vi "View DI param_1.vi"(7 "ActivateDIView":bool, 9 "DI":T1, 10 "DI_State":T3[](array[typedef]), 11 "DI":bool[](array[boolean])) -> (2 "Reread out":bool)   [LabVIEW 2019, in "Inputs.lvlib"]
uses:
  Inputs.lvlib
  Ctl/Parameter State.ctl
  Ctl/DI.ctl
  Ctl/DI short.ctl
  Database/Progress.vi
  Database/PostgreSQL.lvlib
  Logik/Logik.lvlib
panel:
  out "DI9":bool
  out "DI8":bool
  out "DI7":bool
  out "DI6":bool
  out "DI5":bool
  out "DI4":bool
  out "DI3":bool
  out "DI2":bool
  out "DI1":bool
  out "DI0":bool
  out "DI progress":i32(slide) scale=0.0..100.0
  in  "Reread":bool
  in  "n_elem":i32(c297)
  out "n param":i32
  out "Names table":string[](array[string])
  out "parameters":string[](array[string])
  out "Parameters":dbl[][](array[numeric])
  # "module_num"
  # "invert"
  # "time const"
  # "channel_num"
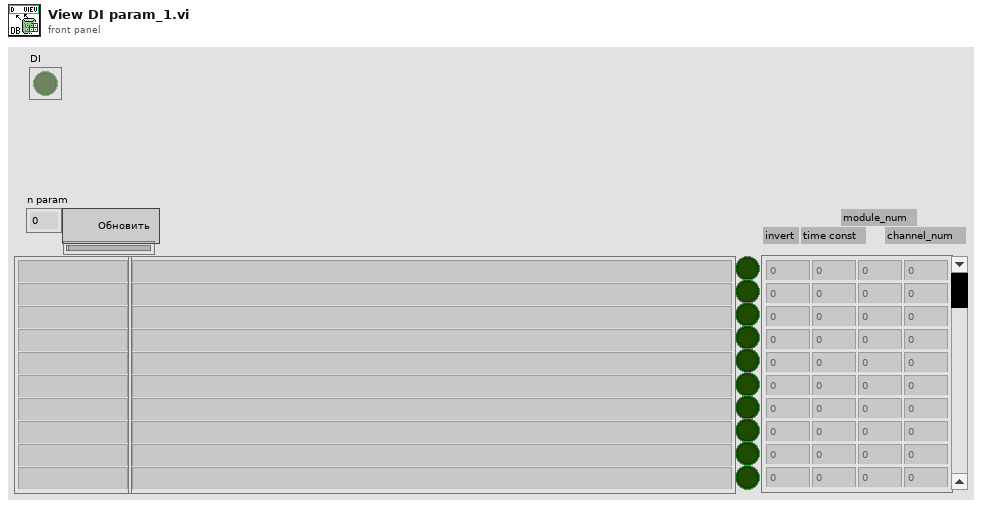
[diagram p1: front panel]
types:
  T1 = typedef "Inputs.lvlib/DI.ctl" = cluster{"DI_defs":T2, "modified":refnum<data-value>, "DIP":refnum<data-value>, "DINames":refnum<data-value>}
  T2 = typedef "Inputs.lvlib/DI short.ctl" = cluster{"DI":bool[], "DI_State":T3[], "DI_ALRState":errorcluster[]}
  T3 = typedef "Inputs.lvlib/Parameter State.ctl" = cluster{"code":i32, "visible":bool, "color":u32, "source":string}
  T4 = enum32{"Invalid", "Standard", "Closed", "Hidden", "Minimized", "Maximized"}
  T5 = enum8{"Enabled", "Disabled", "Disabled and Grayed Out"}
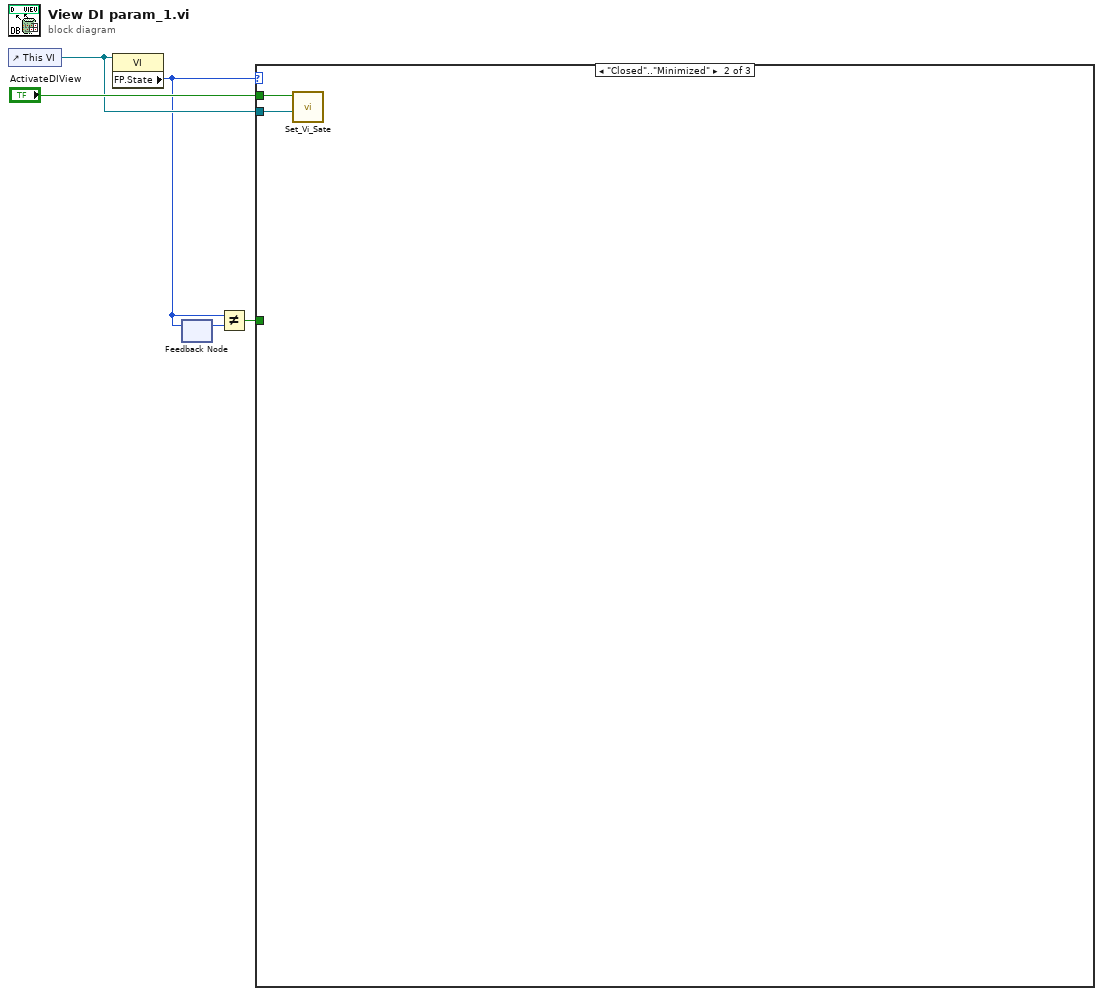
[diagram p0: block diagram]
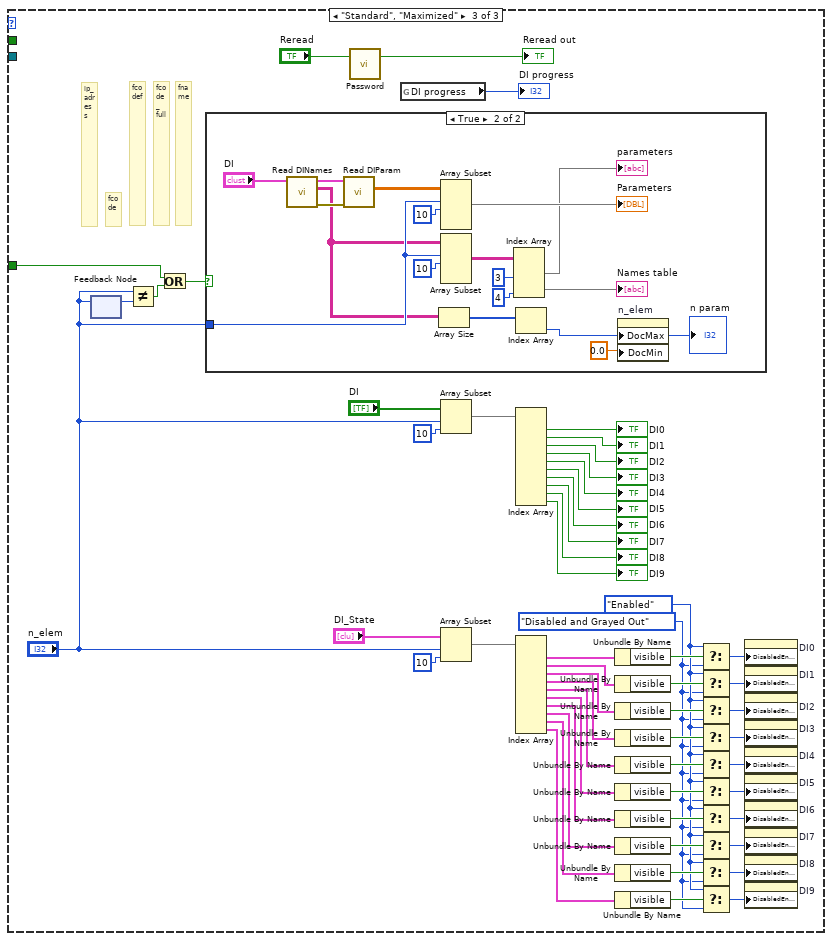
[diagram p3: hidden frame]
diagram:
  n1 = control-ref of="This VI"() -> (w4:refnum<vi>)
  n2 = property class="VI"(reference=w4) -> ("FP.State"=w2:T4)  [unwired: 1 in, 2 out]
  n3 = feedback #1() -> (w3:T4)  [unwired: 1 in]
  n4 = feedback-in #1(w2) -> ()
  n5 = Not Equal?(x=w2, y=w3) -> (x != y?=w1:bool)
  n6 = case shown="\"Closed\"..\"Minimized\"" w2 {
    tunnel: "ActivateDIView" -> [_ w7 _]
    tunnel: w4 -> [_ w6 _]
    tunnel: w1 -> [_ _ w9]
    frame "Invalid", Default {
    }
    frame "Closed".."Minimized" {
      n7 = call "Set_Vi_Sate.vi"("VI"=w6, "Activate (F)"=w7) -> ()  [unwired: 9 in, 1 out]
    }
    frame "Standard", "Maximized" {
      w14 = T5."Enabled" ("Disabled")
      w13 = T5."Disabled and Grayed Out" ("Disabled")
      # "fcode_full"
      # "ip_adress"
      # "fname"
      # "fcodef"
      # "fcode"
      n8 = feedback #2() -> (w11:i32)  [unwired: 1 in]
      n9 = feedback-in #2("n_elem") -> ()
      n10 = Not Equal?(x="n_elem", y=w11) -> (x != y?=w12:bool)
      n11 = Or(x=w9, y=w12) -> (x .or. y?=w8:bool)
      n12 = case shown="True" w8 {
        tunnel: "n_elem" -> [_ w76]
        frame False {
        }
        frame True {
          n13 = call "Read DINames.vi"("DI in"="DI") -> ("error out"=w68:errorcluster, "DINames"=w65:string[][], "DI out"=w67:T1)  [unwired: 8 in]
          n14 = call "Read DIParam.vi"("error in (no error)"=w68, "DI in"=w67) -> ("DIParam"=w66:dbl[][])  [unwired: 7 in, 2 out]
          n15 = Array Size(array=w65) -> (size(s)=w70:i32[])
          n16 = Array Subset(array=w66, index (row)=w76, length (row)=10 ("length")) -> (→"Parameters":dbl[][])  [unwired: 2 in]
          n17 = Array Subset(array=w65, index (row)=w76, length (row)=10 ("length")) -> (w75:string[][])  [unwired: 2 in]
          n18 = Index Array(array=w75, index (col) #1=3 ("length"), index (col) #2=4 ("length")) -> (element #1=→"parameters":string[], element #2=→"Names table":string[])  [unwired: 2 in]
          n19 = Index Array(array=w70) -> (element=w69:i32)  [unwired: 1 in]
          "n param" <- w69
          n20 = property on="n_elem" class="Scroll (strict)"("DocMax"=w69, "DocMin"=0.0 ("Data Entry Limits:Minimum")) -> ()  [unwired: 2 in, 2 out]
        }
      }
      n21 = call "Password.vi"("ActivatePASSWView"="Reread") -> ("enable"=→"Reread out":bool)  [unwired: 1 in, 1 out]
      n22 = global read "Progress.vi" "DI progress"() -> (→"DI progress":i32)
      n23 = Array Subset(array="DI", index="n_elem", length=10) -> (w58:bool[])
      n24 = Array Subset(array="DI_State", index="n_elem", length=10) -> (w45:T3[])
      n25 = Index Array(array=w58) -> (element #1=→"DI0":bool, element #2=→"DI1":bool, element #3=→"DI2":bool, element #4=→"DI3":bool, element #5=→"DI4":bool, element #6=→"DI5":bool, element #7=→"DI6":bool, element #8=→"DI7":bool, element #9=→"DI8":bool, element #10=→"DI9":bool)  [unwired: 10 in]
      n26 = Index Array(array=w45) -> (element #1=w44:T3, element #2=w15:T3, element #3=w16:T3, element #4=w17:T3, element #5=w18:T3, element #6=w19:T3, element #7=w20:T3, element #8=w21:T3, element #9=w22:T3, element #10=w23:T3)  [unwired: 10 in]
      n27 = Unbundle By Name(w44) -> ("visible"=w43:bool)
      n28 = Unbundle By Name(w15) -> ("visible"=w40:bool)
      n29 = Unbundle By Name(w16) -> ("visible"=w39:bool)
      n30 = Unbundle By Name(w17) -> ("visible"=w36:bool)
      n31 = Unbundle By Name(w18) -> ("visible"=w35:bool)
      n32 = Unbundle By Name(w19) -> ("visible"=w32:bool)
      n33 = Unbundle By Name(w20) -> ("visible"=w31:bool)
      n34 = Unbundle By Name(w21) -> ("visible"=w29:bool)
      n35 = Unbundle By Name(w22) -> ("visible"=w27:bool)
      n36 = Unbundle By Name(w23) -> ("visible"=w26:bool)
      n37 = Select(t=w14, s=w43, f=w13) -> (s? t:f=w42:T5)
      n38 = Select(t=w14, s=w40, f=w13) -> (s? t:f=w41:T5)
      n39 = Select(t=w14, s=w39, f=w13) -> (s? t:f=w38:T5)
      n40 = Select(t=w14, s=w36, f=w13) -> (s? t:f=w37:T5)
      n41 = Select(t=w14, s=w35, f=w13) -> (s? t:f=w34:T5)
      n42 = Select(t=w14, s=w32, f=w13) -> (s? t:f=w33:T5)
      n43 = Select(t=w14, s=w31, f=w13) -> (s? t:f=w30:T5)
      n44 = Select(t=w14, s=w29, f=w13) -> (s? t:f=w28:T5)
      n45 = Select(t=w14, s=w27, f=w13) -> (s? t:f=w25:T5)
      n46 = Select(t=w14, s=w26, f=w13) -> (s? t:f=w24:T5)
      n47 = property on="DI0" class="Bool (strict)"("DisabledEnum"=w42) -> ()  [unwired: 2 in, 2 out]
      n48 = property on="DI1" class="Bool (strict)"("DisabledEnum"=w41) -> ()  [unwired: 2 in, 2 out]
      n49 = property on="DI2" class="Bool (strict)"("DisabledEnum"=w38) -> ()  [unwired: 2 in, 2 out]
      n50 = property on="DI3" class="Bool (strict)"("DisabledEnum"=w37) -> ()  [unwired: 2 in, 2 out]
      n51 = property on="DI4" class="Bool (strict)"("DisabledEnum"=w34) -> ()  [unwired: 2 in, 2 out]
      n52 = property on="DI5" class="Bool (strict)"("DisabledEnum"=w33) -> ()  [unwired: 2 in, 2 out]
      n53 = property on="DI6" class="Bool (strict)"("DisabledEnum"=w30) -> ()  [unwired: 2 in, 2 out]
      n54 = property on="DI7" class="Bool (strict)"("DisabledEnum"=w28) -> ()  [unwired: 2 in, 2 out]
      n55 = property on="DI8" class="Bool (strict)"("DisabledEnum"=w25) -> ()  [unwired: 2 in, 2 out]
      n56 = property on="DI9" class="Bool (strict)"("DisabledEnum"=w24) -> ()  [unwired: 2 in, 2 out]
    }
  }
